vi "New Main Log Loop.vi"(8 "error in (no error)":errorcluster) -> (0 "error out":errorcluster)   [LabVIEW 2015]
uses:
  Packet Types.ctl
  Sprocket/src/Refname/Actuators.ctl
  <vilib>/Rock Robotics/WPI/Utilities/WPI_GetSetVariantRefNum.vi
  Main/Robot Global Data.vi
  <vilib>/Rock Robotics/WPI/Solenoid/Deprecated/WPI_SolenoidGetBool.vi
  Sprocket/lib/Sprocket.lvlib
panel:
  out "result string":string
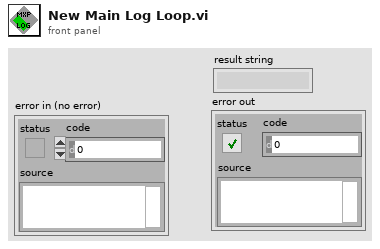
[diagram p1: front panel]
types:
  T1 = typedef "Sprocket.lvlib/Actuators.ctl" = enum16{"Drive Motor 1 (R)", "Drive Motor 2 (R)", "Drive Motor 3 (R)", "Drive Motor 4 (L)", "Drive Motor 5 (L)", "Drive Motor 6 (L)", "Collector Motor", "Collector Solenoid", "Compressor", "SonicShifter", "Gyro", "UltraSonic Front Left", "UltraSonic Back Left", "Wedge Motor", "Wedge LS"}
  T2 = typedef "packet types.ctl" = enum16{"Log line", "Open File", "Send Header", "Set Time", "Send to LCD"}
  T3 = typedef "Packet Types.ctl" = enum16{"Log line", "Open File", "Send Header", "Set Time", "Send to LCD"}
  T4 = typedef "WPI_SerialPortRef.ctl" = cluster{"DevStatus":errorcluster, "Serial Port Name":refnum<visa-resource-name>}
  T5 = typedef "WPI_MotorControlDeviceRef.ctl" = cluster{"DeviceStatus":errorcluster, "Type":T6, "PWM":cluster{"PWM Channel":T7, "DeadBand":T8}, "CAN":cluster{"Device Number":u8, "Control Mode":T9, "Semaphore":T10, "Max Vout":dbl, "TalonSRX Control Mode":T11}, "Invert":bool}
  T6 = typedef "WPI_MotorControlType.ctl" = enum16{"PWM", "CAN", "CANTalonSRX"}
  T7 = typedef "FPGA_DIOPWMChannel.ctl" = enum8{"PWM 0", "PWM 1", "PWM 2", "PWM 3", "PWM 4", "PWM 5", "PWM 6", "PWM 7", "PWM 8", "PWM 9", "PWM MXP 0", "PWM MXP 1", "PWM MXP 2", "PWM MXP 3", "PWM MXP 4", "PWM MXP 5", "PWM MXP 6", "PWM MXP 7", "PWM MXP 8", "PWM MXP 9", "Invalid"}
  T8 = typedef "WPI_PWMDeadband.ctl" = cluster{"Name":string, "maxPositivePwm":i32, "minPositivePwm":i32, "centerPwm":i32, "maxNegativePwm":i32, "minNegativePwm":i32, "angularRange":u16}
  T9 = typedef "WPI_CANJaguar_ControlMode.ctl" = enum8{"Percent VBus", "Current", "Speed", "Position", "Voltage"}
  T10 = typedef "Semaphore RefNum" = refnum<k1>
  T11 = typedef "WPI_CANTalonSRX_APIControlMode.ctl" = enum8{"Percent VBus", "Speed", "Position", "Slave", "Unchanged / Invalid", "Voltage Compensation", "Current", "Motion Profile"}
  T12 = typedef "WPI_CompressorDevRef.ctl" = cluster{"DevStatus":errorcluster, "Pneumatics Control Module":u8}
  T13 = typedef "WPI_SolenoidDevRef.ctl" = cluster{"DevStatus":errorcluster, "Pneumatics Control Module":u8, "Forward Solenoid Channel":T14, "Reverse Solenoid Channel":T14}
  T14 = typedef "WPI_SolenoidChannel.ctl" = enum8{"Solenoid 0", "Solenoid 1", "Solenoid 2", "Solenoid 3", "Solenoid 4", "Solenoid 5", "Solenoid 6", "Solenoid 7", "Invalid"}
  T15 = typedef "WPI_DriverStationRobotMode2.ctl" = enum16{"Autonomous Disabled", "Autonomous Enabled", "Teleop Disabled", "Teleop Enabled", "Disconnected", "Finish", "Test Disabled", "Test Enabled", "Emergency Stopped"}
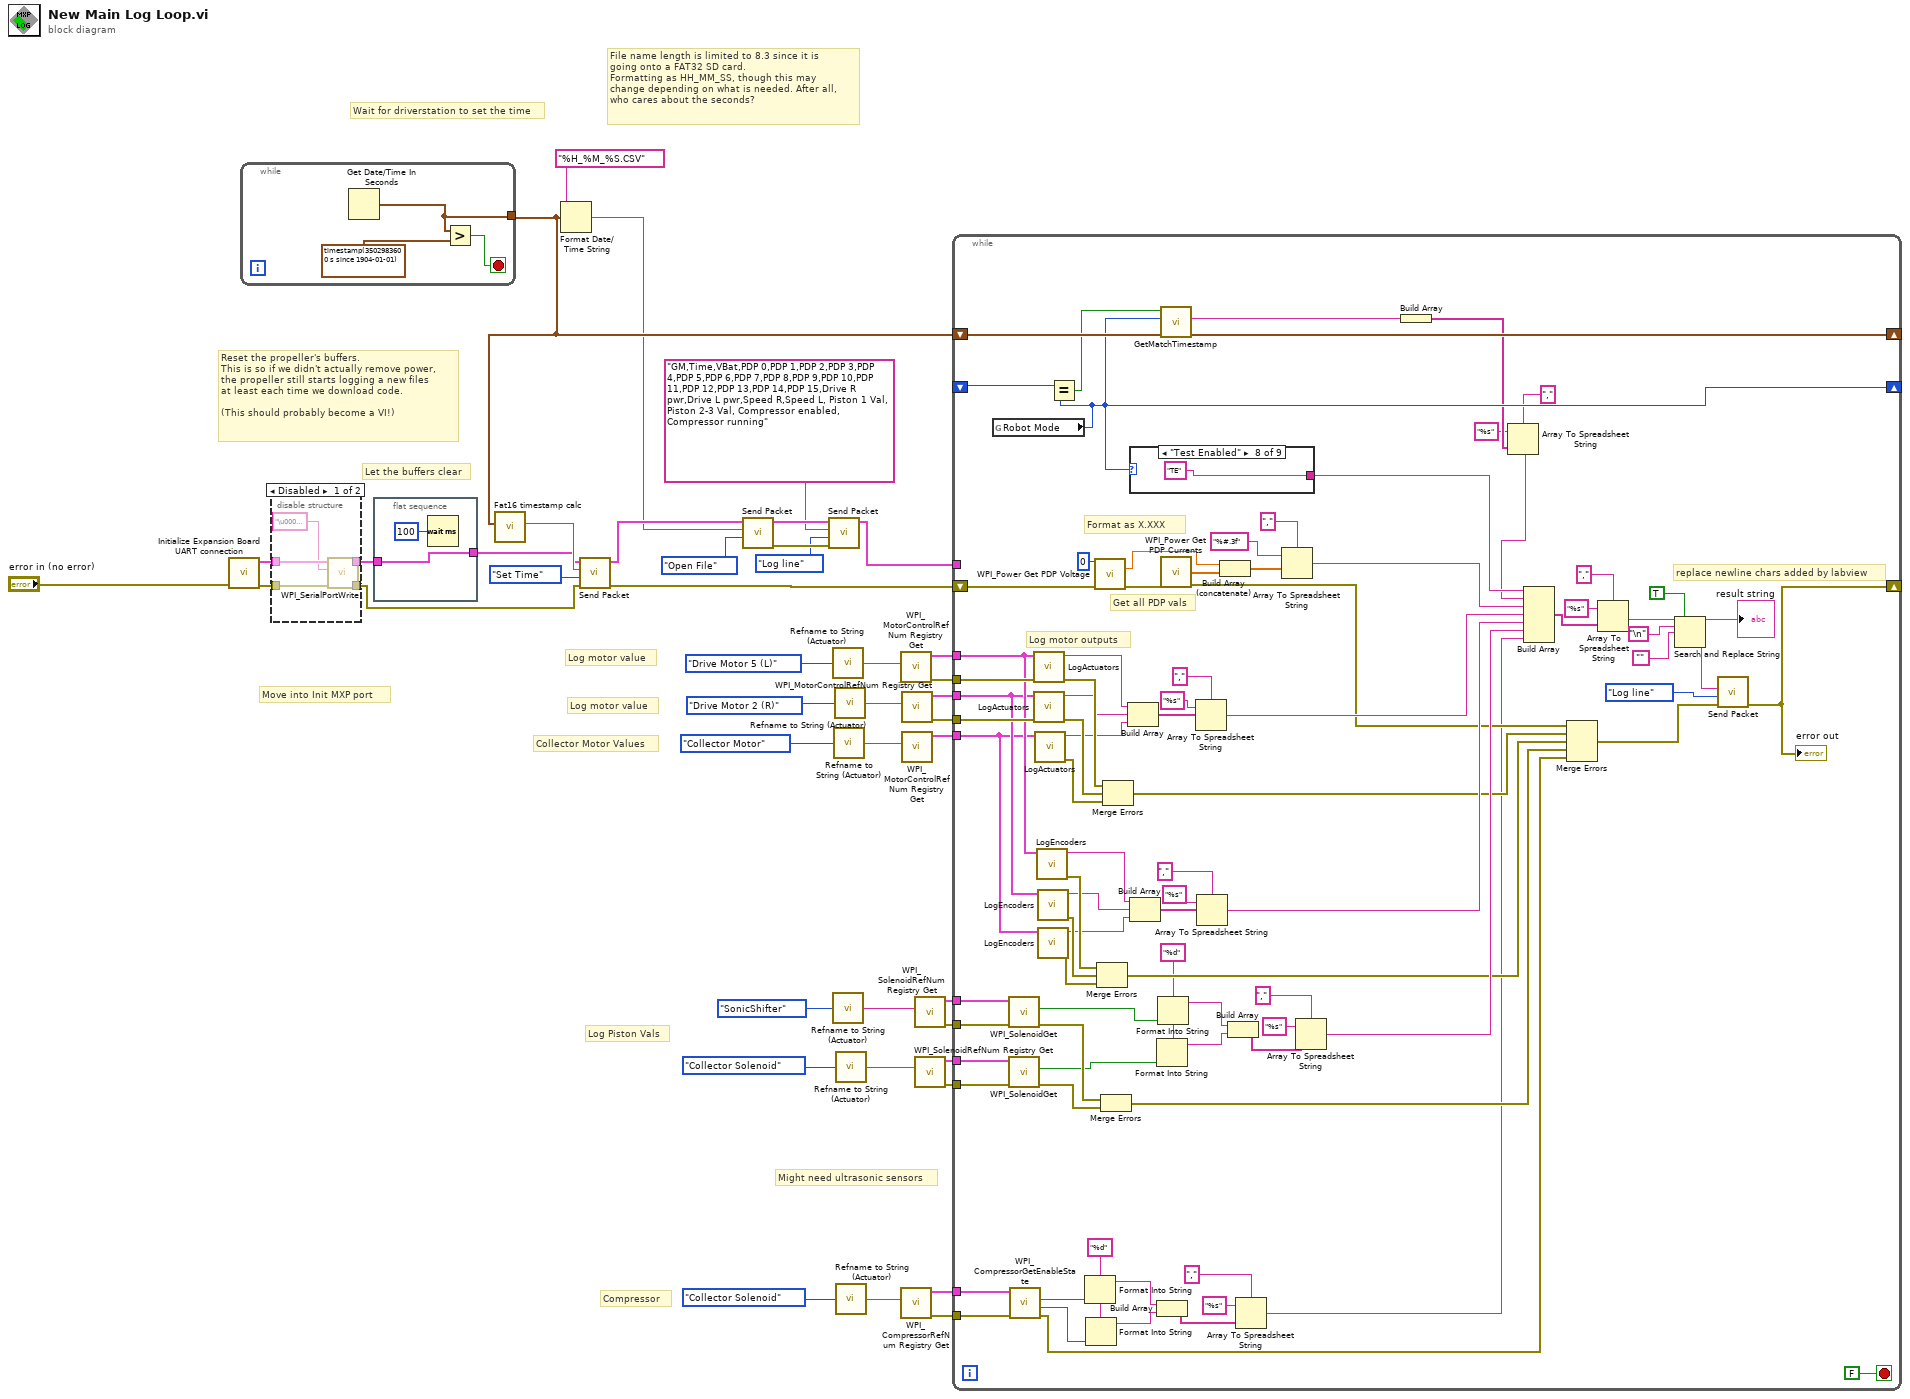
[diagram p0: block diagram]
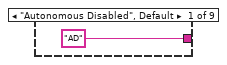
[diagram p2: hidden frame]
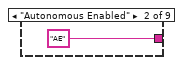
[diagram p3: hidden frame]
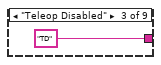
[diagram p4: hidden frame]
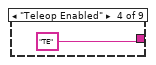
[diagram p5: hidden frame]
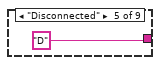
[diagram p6: hidden frame]
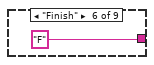
[diagram p7: hidden frame]
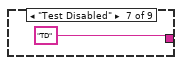
[diagram p8: hidden frame]
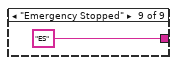
[diagram p9: hidden frame]
diagram:
  # "Might need ultrasonic sensors"
  # "Collector Motor Values"
  # "Compressor"
  # "Log motor value"
  # "Log motor value"
  # "Log Piston Vals"
  # "Move into Init MXP port"
  # "Let the buffers clear"
  # "Reset the propeller's buffers.\nThis is so if we didn't actually remove power,\nthe propeller still starts logging a new files \nat least each time we download code.\n\n(This should probably become a VI!)"
  # "File name length is limited to 8.3 since it is \ngoing onto a FAT32 SD card. \nFormatting as HH_MM_SS, though this may\nchange depending on what is needed. After all,\nwho cares about the seconds?"
  # "Wait for driverstation to set the time"
  n1 = call "Initialize Expansion Board UART connection.vi"("error in (no error)"="error in (no error)") -> ("error out"=w39:errorcluster, "SerialPortRef"=w38:T4)  [unwired: 9 in]
  n2 = while {
    tunnel: [w43] -> w33
    stop <- w44 stop-if-true
    n3 = Get Date/Time In Seconds() -> (seconds since 1Jan1904=w43:timestamp)
    n4 = Greater?(x=w43, y=timestamp(3502983600 s since 1904-01-01)) -> (0:w44:bool)
  }
  n5 = disable-structure shown="Disabled" {
    disable-tunnel: w39 -> [w50 w51]
    disable-tunnel: w38 -> [w49 w52]
    disable-tunnel: [w47 w52] -> w36
    disable-tunnel: [w46 w51] -> w35
    frame Disabled {
      n6 = call <vilib>:"WPI_SerialPortWrite.vi"("error in (no error)"=w50, "Buffer"="\u0004\u0004", "SerialPortRef"=w49) -> ("error out"=w46:errorcluster, "SerialPortRef"=w47:T4)  [unwired: 6 in, 1 out]
    }
    frame Enabled {
    }
  }
  n7 = flat-sequence {
    tunnel: [w54] -> w37
    tunnel: w36 -> [w54]
    frame #0 {
      n8 = Wait (ms)(milliseconds to wait=u32 100) -> ()  [unwired: 1 out]
    }
  }
  n9 = call "Fat16 timestamp calc.vi"("time stamp"=w33) -> ("timestamp as string"=w41:string)  [unwired: 10 in]
  n10 = Format Date/Time String(time format string (%c)="%H_%M_%S.CSV", seconds (now)=w33) -> (date/time string=w26:string)  [unwired: 1 in]
  n11 = call "Send Packet.vi"("error in (no error)"=w35, 7:Packet_Types."Set Time", "Log string"=w41, "SerialPortRef"=w37) -> ("error out"=w24:errorcluster, "SerialPortRef out"=w27:T4)  [unwired: 4 in]
  n12 = call "Send Packet.vi"(7:packet_types."Open File", "Log string"=w26, "SerialPortRef"=w27) -> ("error out"=w31:errorcluster, "SerialPortRef out"=w32:T4)  [unwired: 5 in]
  n13 = call "Send Packet.vi"("error in (no error)"=w31, 7:packet_types."Log line", "Log string"="GM,Time,VBat,PDP 0,PDP 1,PDP 2,PDP 3,PDP 4,PDP 5,PDP 6,PDP 7,PDP 8,PDP 9,PDP 10,PDP 11,PDP 12,PDP 13,PDP 14,PDP 15,Drive R pwr,Drive L pwr,Speed R,Speed L, Piston 1 Val, Piston 2-3 Val, Compressor enabled, Compressor running", "SerialPortRef"=w32) -> ("SerialPortRef out"=w28:T4)  [unwired: 4 in, 1 out]
  n14 = call "Refname to String (Actuator).vi"("Actuator Refname"=Actuators."Drive Motor 5 (L)") -> ("Refnum Name"=w21:string)
  n15 = call "Refname to String (Actuator).vi"("Actuator Refname"=Actuators."SonicShifter") -> ("Refnum Name"=w11:string)
  n16 = call "Refname to String (Actuator).vi"("Actuator Refname"=Actuators."Collector Motor") -> ("Refnum Name"=w14:string)
  n17 = call "Refname to String (Actuator).vi"("Actuator Refname"=Actuators."Drive Motor 2 (R)") -> ("Refnum Name"=w19:string)
  n18 = call "Refname to String (Actuator).vi"("Actuator Refname"=Actuators."Collector Solenoid") -> ("Refnum Name"=w7:string)
  n19 = call "Refname to String (Actuator).vi"("Actuator Refname"=Actuators."Collector Solenoid") -> ("Refnum Name"=w2:string)
  n20 = call <vilib>:"WPI_MotorControlRefNum Registry Get.vi"("refnum name"=w21) -> ("error out"=w17:errorcluster, "MotorControlDevRef"=w22:T5)  [unwired: 9 in]
  n21 = call <vilib>:"WPI_CompressorRefNum Registry Get.vi"("refnum name"=w2) -> ("error out"=w1:errorcluster, "CompressorDevRef"=w3:T12)  [unwired: 9 in]
  n22 = call <vilib>:"WPI_MotorControlRefNum Registry Get.vi"("refnum name"=w19) -> ("error out"=w16:errorcluster, "MotorControlDevRef"=w18:T5)  [unwired: 9 in]
  n23 = call <vilib>:"WPI_MotorControlRefNum Registry Get.vi"("refnum name"=w14) -> ("MotorControlDevRef"=w13:T5)  [unwired: 9 in, 1 out]
  n24 = call <vilib>:"WPI_SolenoidRefNum Registry Get.vi"("refnum name"=w11) -> ("error out"=w9:errorcluster, "SolenoidDevRef"=w10:T13)  [unwired: 9 in]
  n25 = call <vilib>:"WPI_SolenoidRefNum Registry Get.vi"("refnum name"=w7) -> ("error out"=w5:errorcluster, "SolenoidDevRef"=w8:T13)  [unwired: 9 in]
  n26 = while {
    shift-right: [w139] -> _
    shift-left: w33 -> [w138]
    shift-right: [w135] -> _
    shift-left: _ -> [w137]
    tunnel: w28 -> [_]
    tunnel: w18 -> [w66]
    tunnel: w8 -> [w108]
    shift-right: [w85] -> _
    shift-left: w24 -> [w84]
    tunnel: w3 -> [w83]
    tunnel: w17 -> [w69]
    tunnel: w22 -> [w67]
    tunnel: w16 -> [w68]
    tunnel: w13 -> [w65]
    tunnel: w10 -> [w64]
    tunnel: w9 -> [w63]
    tunnel: w5 -> [w62]
    tunnel: w1 -> [w59]
    stop <- FALSE stop-if-true
    w55 = "%d" ("format string")
    w56 = "%d" ("format string")
    # "Get all PDP vals"
    # "replace newline chars added by labview"
    # "Log motor outputs"
    # "Format as X.XXX"
    n27 = global read "Robot Global Data.vi" "Robot Mode"() -> (w135:T15)
    n28 = call-poly <vilib>:"WPI_SolenoidGet.vi"("error in (no error)"=w63, "SolenoidDevRef"=w64) -> ("error out"=w106:errorcluster, "Value"=w105:bool)  [unwired: 7 in, 1 out]
    n29 = call-poly <vilib>:"WPI_SolenoidGet.vi"("error in (no error)"=w62, "SolenoidDevRef"=w108) -> ("error out"=w107:errorcluster, "Value"=w104:bool)  [unwired: 7 in, 1 out]
    n30 = call <vilib>:"WPI_CompressorGetEnableState.vi"("error in (no error)"=w59, "CompressorDevRef"=w83) -> ("error out"=w61:errorcluster, "Compressor Running"=w77:bool, "Enabled"=w78:bool)  [unwired: 6 in, 1 out]
    n31 = call "LogActuators.vi"("error in (no error) 2"=w69, "MotorControlDevRef"=w67) -> ("error out"=w116:errorcluster, "resulting string"=w113:string)  [unwired: 8 in]
    n32 = call "LogActuators.vi"("error in (no error) 2"=w68, "MotorControlDevRef"=w66) -> ("error out"=w117:errorcluster, "resulting string"=w112:string)  [unwired: 8 in]
    n33 = call "LogActuators.vi"("MotorControlDevRef"=w65) -> ("error out"=w118:errorcluster, "resulting string"=w111:string)  [unwired: 9 in]
    n34 = call "LogEncoders.vi"("CAN Talon SRX Ref"=w67) -> ("error out"=w142:errorcluster, "concatenated string"=w131:string)  [unwired: 9 in]
    n35 = call "LogEncoders.vi"("CAN Talon SRX Ref"=w66) -> ("error out"=w141:errorcluster, "concatenated string"=w130:string)  [unwired: 9 in]
    n36 = call "LogEncoders.vi"("CAN Talon SRX Ref"=w65) -> ("error out"=w140:errorcluster, "concatenated string"=w129:string)  [unwired: 9 in]
    n37 = Equal?(x=w137, y=w135) -> (x = y?=w136:bool)
    n38 = Format Into String(format string=w55, w78) -> (resulting string=w81:string)  [unwired: 2 in, 1 out]
    n39 = Format Into String(format string=w55, w77) -> (resulting string=w80:string)  [unwired: 2 in, 1 out]
    n40 = call <vilib>:"WPI_Power Get PDP Voltage.vi"("Power Distribution Panel (0)"=u8 0, "error in"=w84) -> ("voltage (V)"=w125:dbl, "error out"=w122:errorcluster)  [unwired: 12 in]
    n41 = Merge Errors(w142, w141, w140) -> (w88:errorcluster)
    n42 = Merge Errors(w106, w107) -> (w87:errorcluster)
    n43 = Merge Errors(w116, w117, w118) -> (w89:errorcluster)
    n44 = Build Array(w113, w112, w111) -> (w115:string[])
    n45 = case shown="\"Test Enabled\"" w135 {
      tunnel: ["AD" "AE" "TD" "TE" "D" "F" "TD" "TE" "ES"] -> w134
      frame "Autonomous Disabled", Default {
      }
      frame "Autonomous Enabled" {
      }
      frame "Teleop Disabled" {
      }
      frame "Teleop Enabled" {
      }
      frame "Disconnected" {
      }
      frame "Finish" {
      }
      frame "Test Disabled" {
      }
      frame "Test Enabled" {
      }
      frame "Emergency Stopped" {
      }
    }
    n46 = Build Array(w131, w130, w129) -> (w133:string[])
    n47 = Format Into String(format string=w56, w104) -> (resulting string=w101:string)  [unwired: 2 in, 1 out]
    n48 = Build Array(w81, w80) -> (w82:string[])
    n49 = Format Into String(format string=w56, w105) -> (resulting string=w102:string)  [unwired: 2 in, 1 out]
    n50 = call "GetMatchTimestamp.vi"("seconds since 1Jan1904"=w138, "Robot Mode"=w135, "Boolean"=w136) -> ("seconds since 1Jan1904 2"=w139:timestamp, "Match Timestamp"=w71:string)  [unwired: 7 in]
    n51 = call <vilib>:"WPI_Power Get PDP Currents.vi"("error in"=w122) -> ("all currents (A)"=w123:dbl[], "error out"=w90:errorcluster)  [unwired: 12 in, 1 out]
    n52 = Array To Spreadsheet String(delimiter (Tab)=",", array=w115, 3:"%s" ("format string")) -> (spreadsheet string=w109:string)
    n53 = Array To Spreadsheet String(delimiter (Tab)=",", array=w133, 3:"%s" ("format string")) -> (spreadsheet string=w110:string)
    n54 = Build Array (concatenate)(w125, w123) -> (w124:dbl[])
    n55 = Build Array(w102, w101) -> (w103:string[])
    n56 = Array To Spreadsheet String(delimiter (Tab)=",", array=w82, 3:"%s" ("format string")) -> (spreadsheet string=w60:string)
    n57 = Array To Spreadsheet String(delimiter (Tab)=",", array=w124, 3:"%#.3f" ("format string")) -> (spreadsheet string=w121:string)
    n58 = Array To Spreadsheet String(delimiter (Tab)=",", array=w103, 3:"%s" ("format string")) -> (spreadsheet string=w99:string)
    n59 = Build Array(w71) -> (w70:string[])
    n60 = Array To Spreadsheet String(delimiter (Tab)=",", array=w70, 3:"%s" ("format string")) -> (spreadsheet string=w120:string)
    n61 = Build Array(w134, w120, w121, w109, w110, w99, w60) -> (w93:string[])
    n62 = Merge Errors(w90, w89, w88, w87, w61) -> (w86:errorcluster)
    n63 = Array To Spreadsheet String(delimiter (Tab)=",", array=w93, 3:"%s" ("format string")) -> (spreadsheet string=w94:string)
    n64 = Search and Replace String(replace all?=TRUE ("replace all? (F)"), input string=w94, search string="\n", replace string="") -> (result string=w92:string)  [unwired: 4 in, 3 out]
    "result string" <- w92
    n65 = call "Send Packet.vi"("error in (no error)"=w86, 7:packet_types."Log line", "Log string"=w92) -> ("error out"=w85:errorcluster)  [unwired: 5 in, 1 out]
    "error out" <- w85
  }
